vi "Actor Core.vi"(8 "error in":errorcluster, 11 "Test Info in":refnum<class "Test Info.lvclass">) -> (0 "error out":errorcluster, 3 "Actor out":refnum<class "Actor.lvclass">)   [LabVIEW 2023, in "Data Analysis.lvlib" / "Test Info.lvlib" / "Test Info.lvclass"]
doc: "(<B>Filename</B>: Actor Framework.lvlib:Actor.lvclass:Actor Core.vi)\n\nReceives messages to the actor, reacts to them, and initiates any error handling that may shut the actor down.\n\nDescendant classes may override this VI to append parallel tasks for the actor to complete while it handles messages. Overrides use the Call Parent Class Method node."
uses:
  Test Info.lvclass
  <vilib>/ActorFramework/Actor/Actor.lvclass
  Test Info.lvclass/Test Info.ctl
  <vilib>/ActorFramework/Actor/Actor.lvclass/Actor.ctl
  <vilib>/ActorFramework/Message Enqueuer/Message Enqueuer.lvclass/Message Enqueuer.ctl
  Subpanel-Abstract Messages/Insert SP Msg/Insert SP Msg.lvclass/Insert SP Msg.ctl
  Test Info Messages/Test Log Schema Update Msg/Test Log Schema Update Msg.lvclass/Test Log Schema Update Msg.ctl
  <vilib>/ActorFramework/Message Enqueuer/Init from Existing Queue.vi
  <vilib>/ActorFramework/Message Enqueuer/Enqueue.vi
  Subpanel-Abstract Messages/Insert SP Msg/Insert SP Msg.lvclass
  Test Info Messages/Test Log Schema Update Msg/Test Log Schema Update Msg.lvclass
  <vilib>/ActorFramework/Message Priority Queue/Priority Enqueue.vi
  <vilib>/ActorFramework/Message Enqueuer/Message Enqueuer.lvclass
  Subpanel-Abstract/Subpanel-Abstract.lvclass
panel:
  out "Completed Time":string
  out "Test Start Date":string
  out "Estimated  Completion Date":string
  out "Cycle Completed":u32
  out "Remaining Time":string
  out "Completed Percentage":dbl format="%#_3g%%"
  out "Total Cycles":u32
  out "Remaining Cycles":u32
  in  "Stop":bool
  in  "Test Info":i32(listbox)=-1 caption="Data"
  # "Test Info"
  # "* No filters are applicable here."
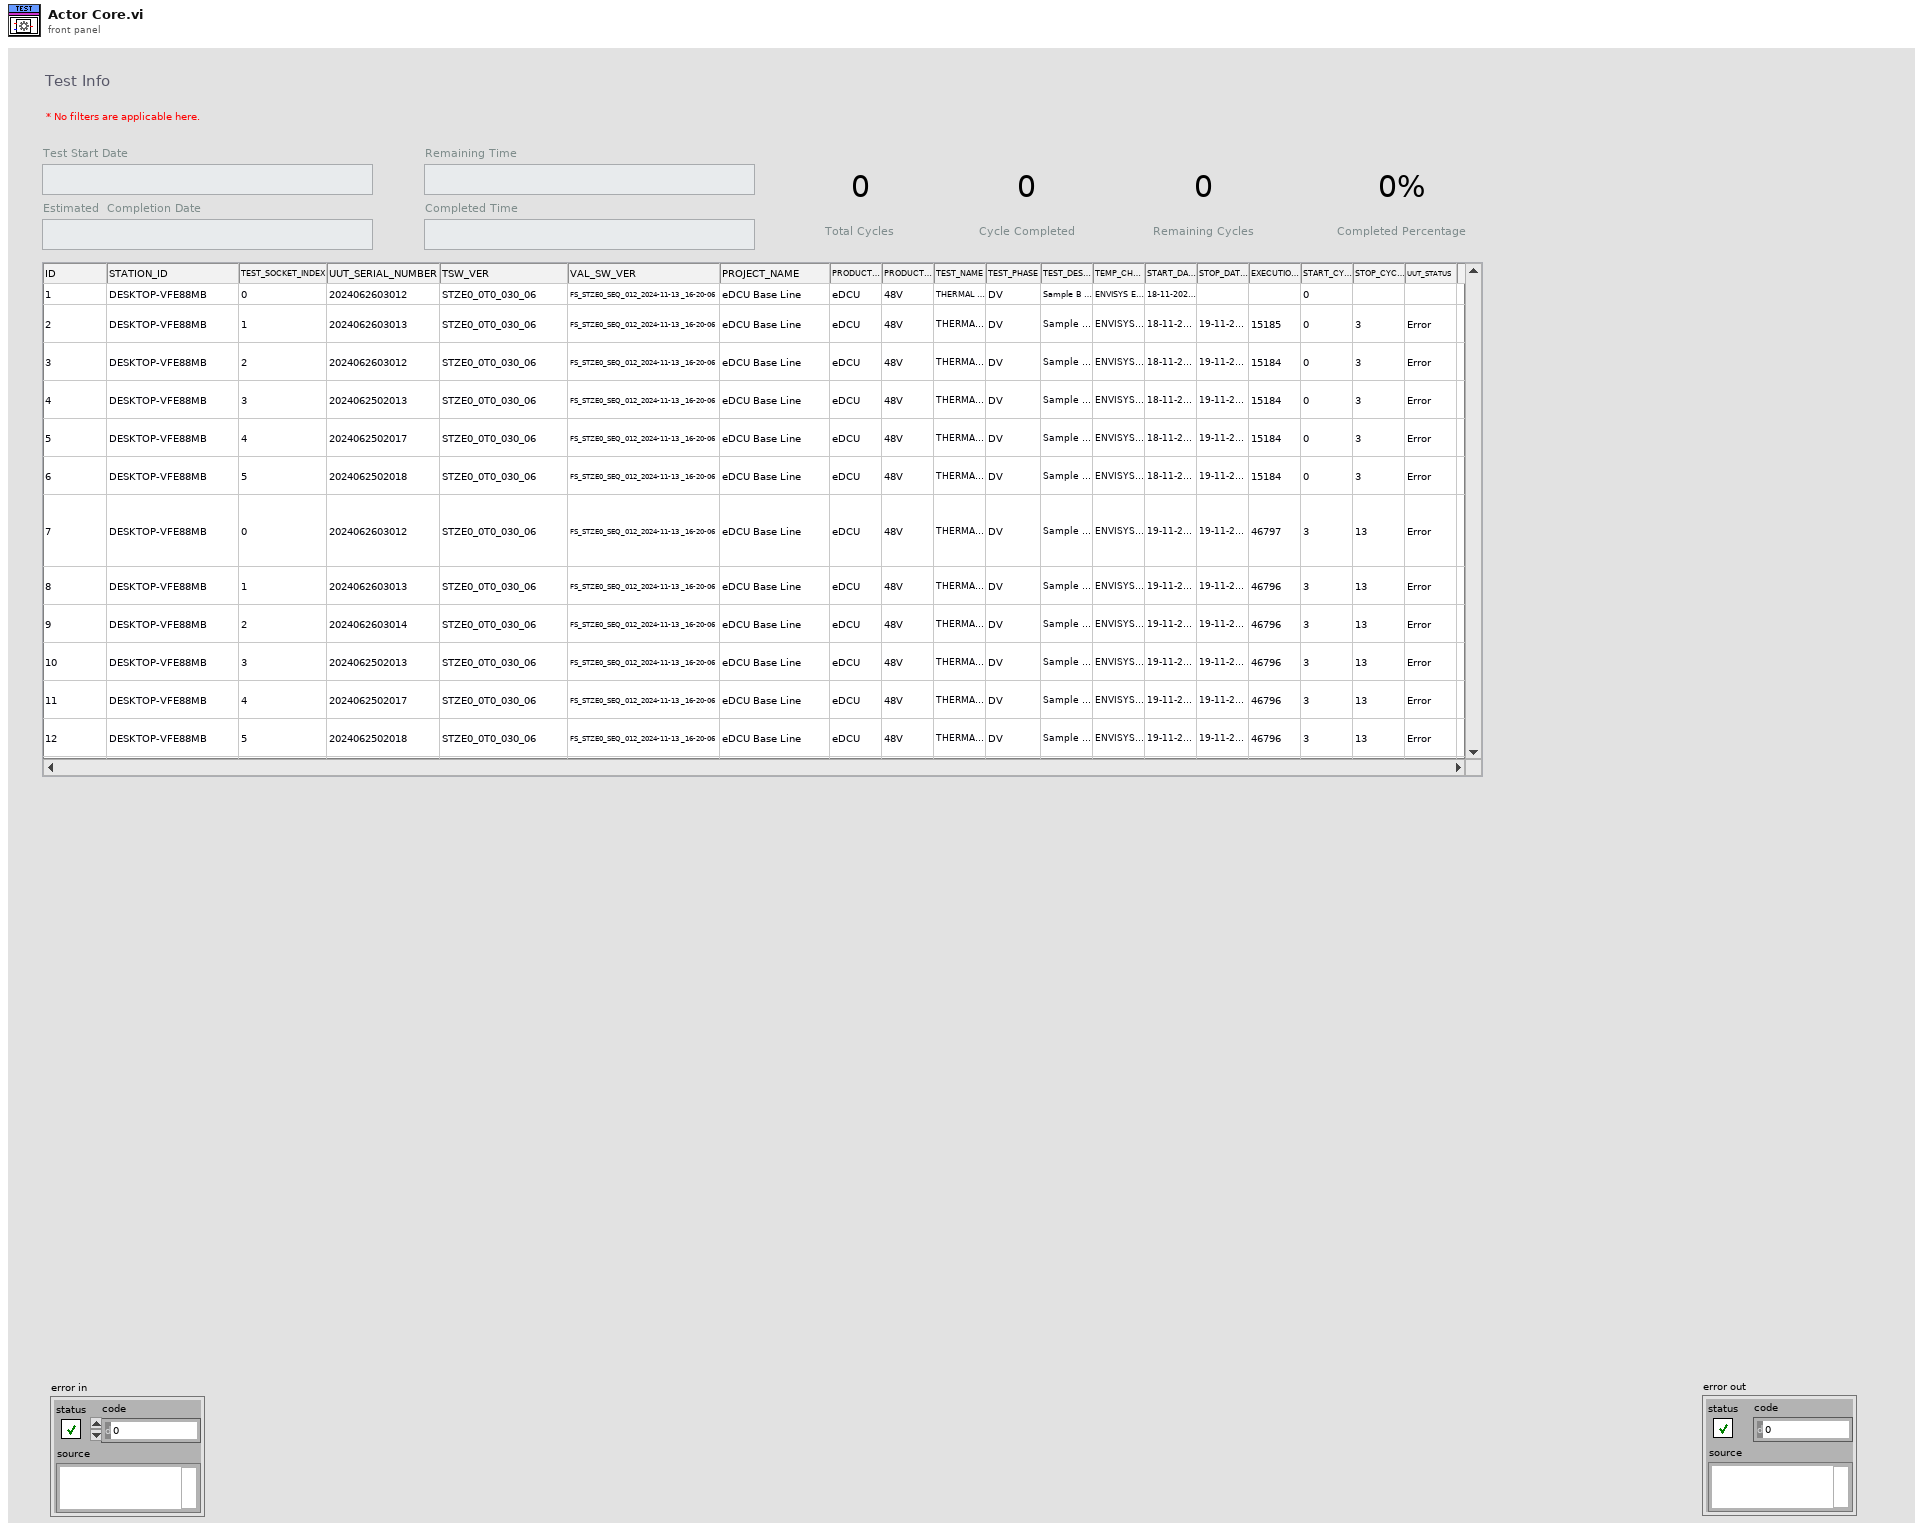
[diagram p1: front panel]
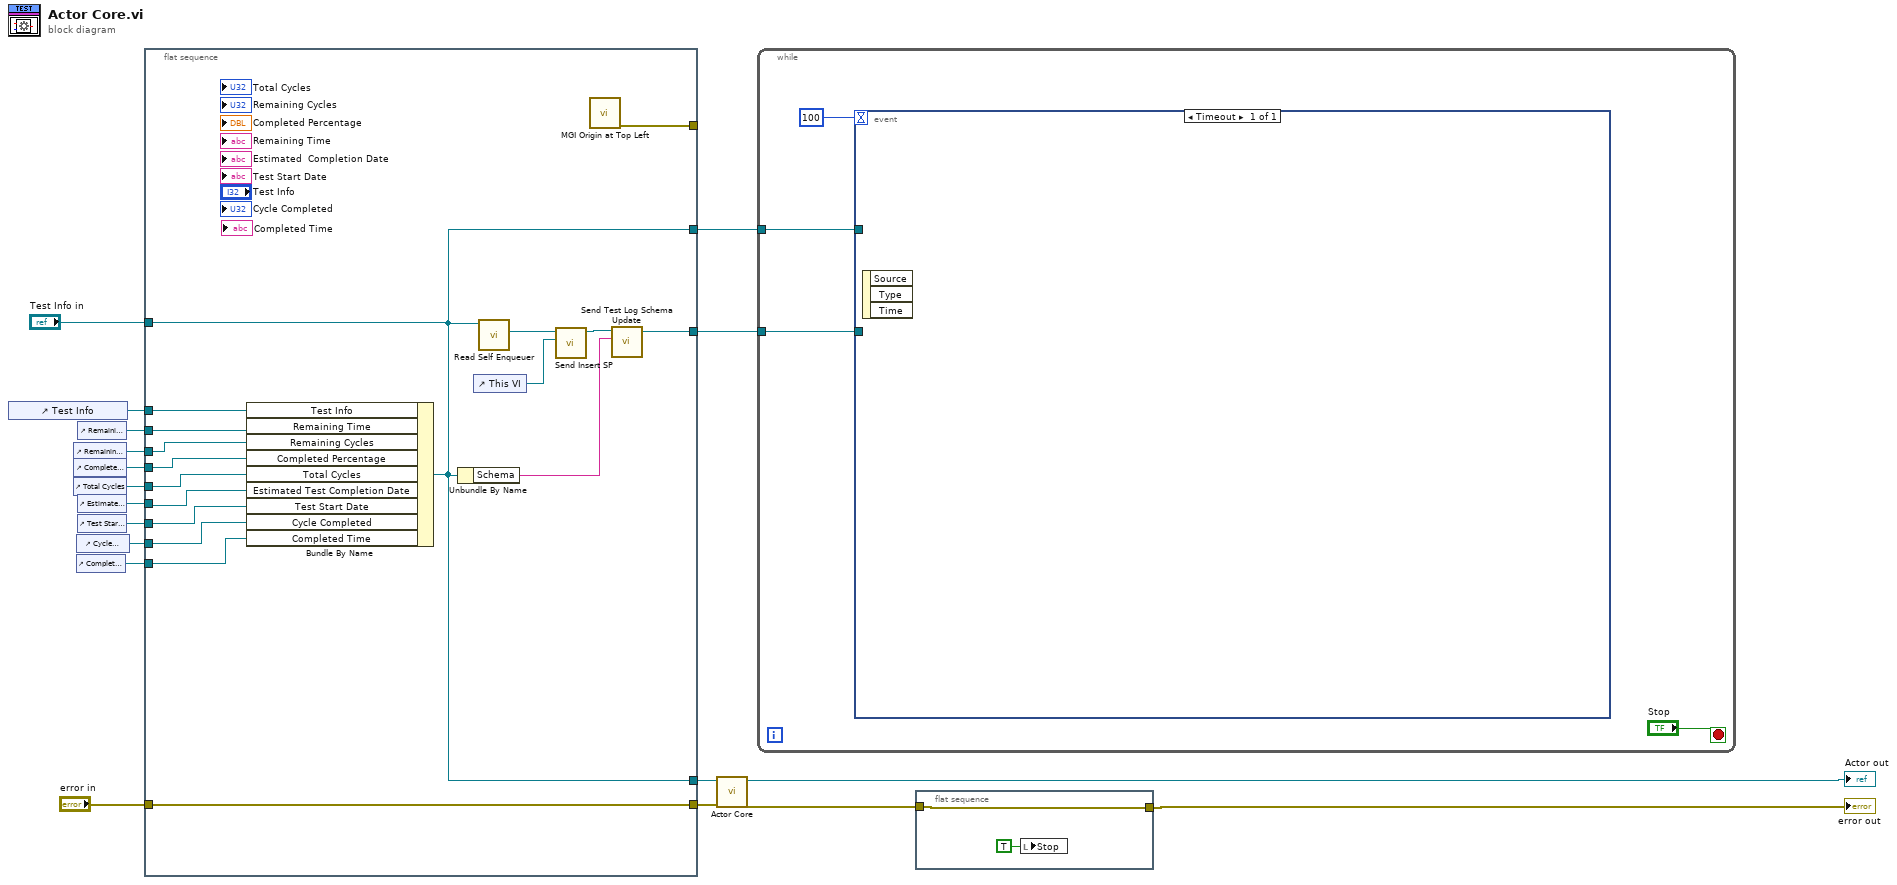
[diagram p0: block diagram]
diagram:
  n1 = control-ref of="Test Info"() -> (w9:refnum<vi>)
  n2 = control-ref of="Remaining Cycles"() -> (w7:refnum<vi>)
  n3 = control-ref of="Completed Percentage"() -> (w6:refnum<vi>)
  n4 = control-ref of="Total Cycles"() -> (w5:refnum<vi>)
  n5 = control-ref of="Cycle Completed"() -> (w2:refnum<vi>)
  n6 = control-ref of="Completed Time"() -> (w1:refnum<vi>)
  n7 = control-ref of="Remaining Time"() -> (w8:refnum<vi>)
  n8 = control-ref of="Estimated  Completion Date"() -> (w4:refnum<vi>)
  n9 = control-ref of="Test Start Date"() -> (w3:refnum<vi>)
  n10 = flat-sequence {
    tunnel: "Test Info in" -> [w32]
    tunnel: [w27] -> w14
    tunnel: "error in" -> [w36]
    tunnel: [w36] -> w12
    tunnel: [w29] -> w11
    tunnel: [w27] -> w10
    tunnel: [w33] -> _
    tunnel: w9 -> [w31]
    tunnel: w8 -> [w26]
    tunnel: w7 -> [w25]
    tunnel: w6 -> [w24]
    tunnel: w5 -> [w23]
    tunnel: w4 -> [w22]
    tunnel: w3 -> [w21]
    tunnel: w2 -> [w20]
    tunnel: w1 -> [w19]
    frame #0 {
      n11 = Bundle By Name(cluster=w32, "Test Info"=w31, "Remaining Time"=w26, "Remaining Cycles"=w25, "Completed Percentage"=w24, "Total Cycles"=w23, "Estimated Test Completion Date"=w22, "Test Start Date"=w21, "Cycle Completed"=w20, "Completed Time"=w19) -> (w27:refnum<class "Test Info.lvclass">)
      n12 = Unbundle By Name(w27) -> ("Schema"=w28:string)
      n13 = control-ref of="This VI"() -> (w34:refnum<vi>)
      n14 = call <vilib>:"Read Self Enqueuer.vi"("Actor"=w27) -> ("Self Enqueuer"=w35:refnum<class "Message Enqueuer.lvclass">)  [unwired: 10 in]
      n15 = call "Send Insert SP.vi"("VI Ref"=w34, "Message Enqueuer"=w35) -> ("Message Enqueuer out"=w30:refnum<class "Message Enqueuer.lvclass">)  [unwired: 8 in, 1 out]
      n16 = call <userlib>:"MGI Origin at Top Left.vi"() -> ("Error Out"=w33:errorcluster)  [unwired: 9 in, 1 out]
      n17 = call "Send Test Log Schema Update.vi"("Schema"=w28, "Message Enqueuer"=w30) -> ("Message Enqueuer out"=w29:refnum<class "Message Enqueuer.lvclass">)  [unwired: 8 in, 1 out]
    }
  }
  n18 = call-parent "Actor Core.vi"("error in"=w12, "Actor in"=w14) -> ("error out"=w17:errorcluster, "Actor out"=→"Actor out":refnum<class "Actor.lvclass">)  [unwired: 8 in]
  n19 = while {
    tunnel: w11 -> [w38]
    tunnel: w10 -> [w37]
    stop <- "Stop" stop-if-true
    n20 = event shown="[0] Timeout" {
      selector: _ -> [_]
      dyn-events: _ -> [_]
      timeout: 100 -> [_]
      tunnel: w38 -> [_]
      tunnel: w37 -> [_]
      event Timeout {
        n21 = event-data() -> ()  [unwired: 1 in, 3 out]
      }
    }
  }
  n22 = flat-sequence {
    tunnel: w17 -> [w42]
    tunnel: [w42] -> w16
    frame #0 {
      n23 = local write "Stop"(TRUE ("Stop")) -> ()
    }
  }
  "error out" <- w16
